vi "TempestAPI.vi"() -> ()   [LabVIEW 2021]
uses:
  <vilib>/httpClient/LabVIEWHTTPClient.lvlib
panel:
  in  "url":string="https://swd.weatherflow.com/swd/rest/observations/device/104016?token=331b6c86-290f-4713-b6a8-f6af7cd94eaa"
  out "body":string
  out "headers":string
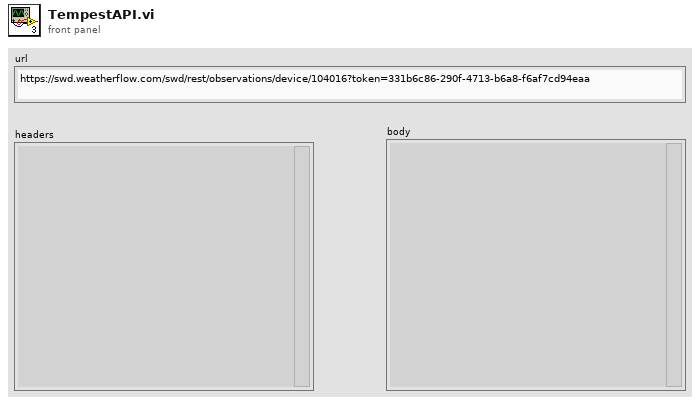
[diagram p1: front panel]
types:
  T1 = typedef "LabVIEWHTTPClient.lvlib/ClientHandle.ctl" = refnum<k1>
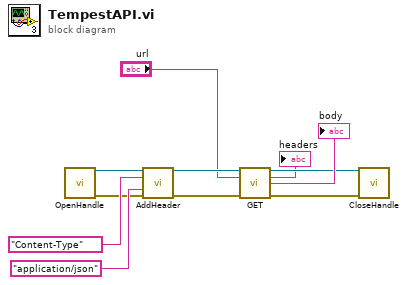
[diagram p0: block diagram]
diagram:
  n1 = call <vilib>:"OpenHandle.vi"() -> ("client handle out"=w7:T1, "error out"=w6:errorcluster)  [unwired: 14 in]
  n2 = call <vilib>:"AddHeader.vi"("client handle"=w7, "header"="Content-Type", "value"="application/json", "error in (no error)"=w6) -> ("client handle out"=w8:T1, "error out"=w9:errorcluster)  [unwired: 10 in]
  n3 = call <vilib>:"GET.vi"("client handle"=w8, "url"="url", "error in (no error)"=w9) -> ("client handle out"=w4:T1, "headers"=→"headers":string, "body"=→"body":string, "error out"=w3:errorcluster)  [unwired: 9 in]
  n4 = call <vilib>:"CloseHandle.vi"("client handle"=w4, "error in (no error)"=w3) -> ()  [unwired: 13 in, 1 out]
